vi "Test.vi"() -> ()   [LabVIEW 2019]
uses:
  <vilib>/NI/Modbus Library/API/Wrapper/Create Serial Master.vi
  <vilib>/NI/Modbus Library/API/Master/Modbus Master.lvclass
  <vilib>/NI/Modbus Library/API/Wrapper/API Main.lvlib
panel:
  in  "register to write":u16=50
  out "read values":u16[](array[numeric])
  in  "read count":u16=1
  in  "read starting address":u16=302 format="%04d"
  out "error out":errorcluster
  out "FTCU Input Reg Value":u16[](array[numeric])
  in  "FTCU Hold Reg Addr":u16=302 format="%04d"
  in  "FTCU Input Reg Addr":u16=8 format="%04d"
  in  "stop":bool
  in  "frequency":u16 caption="frequency, 0.01 Hz"
  in  "address":u16=895 format="%04x"
  in  "number of inputs":u16=1
  in  "starting address":u16=18 format="%04x"
  out "register values":u16[](array[numeric])
  # "G100"
  # "0h037F - adres zadawania prêdkoœci\ntab 7.6.2, str. 236"
  # "2 Hz to minimum"
  # "FTCU"
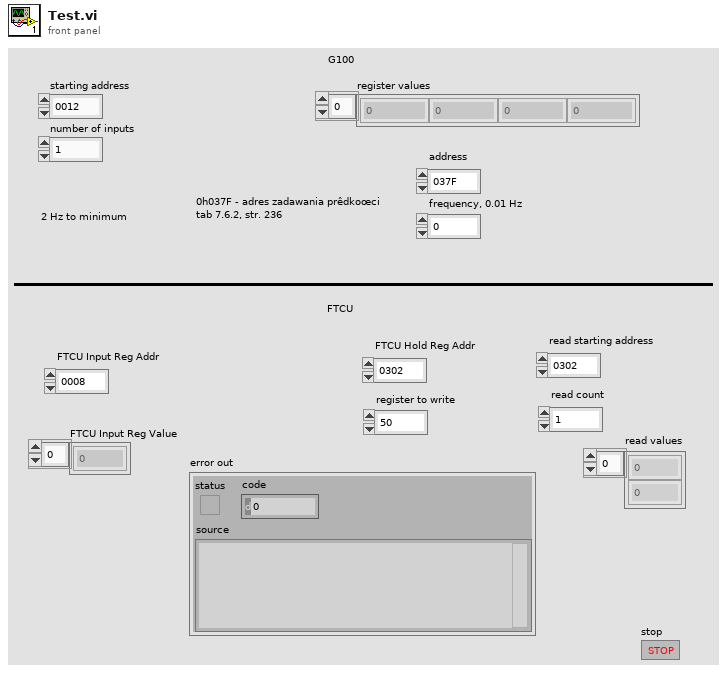
[diagram p1: front panel]
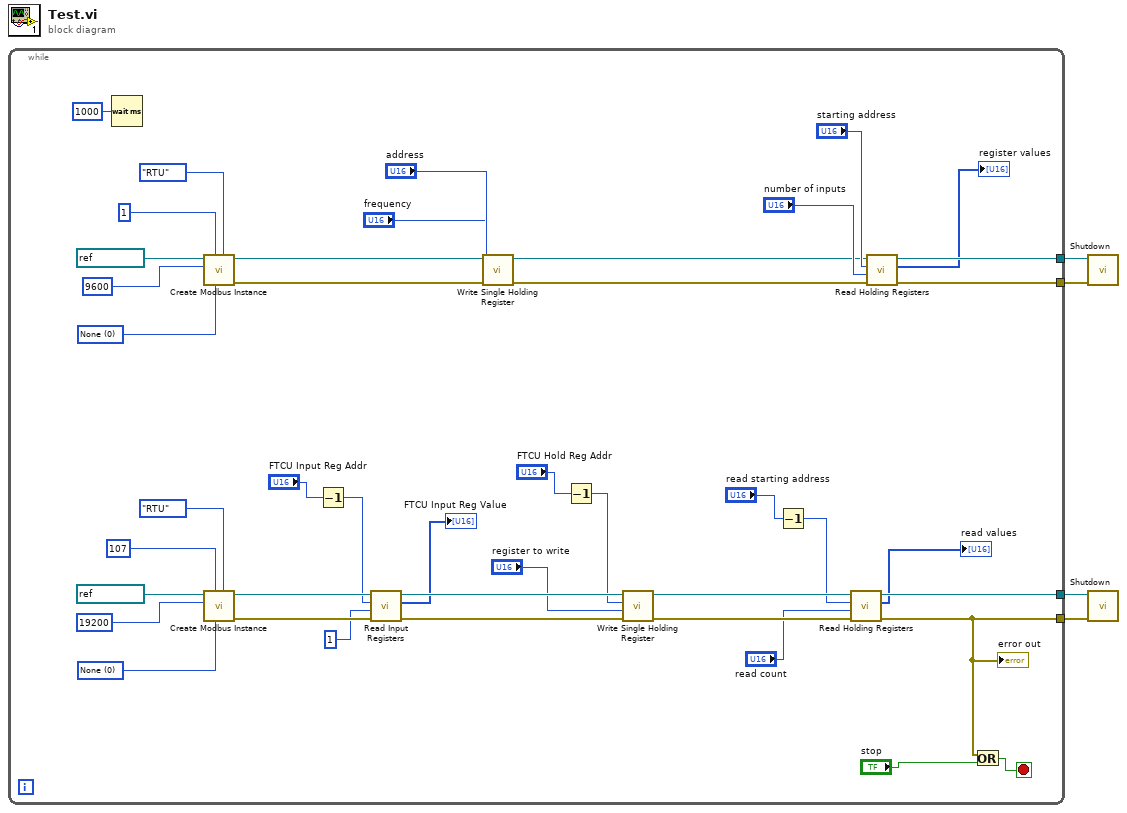
[diagram p0: block diagram]
diagram:
  n1 = while {
    tunnel: [w40] -> w4
    tunnel: [w39] -> w3
    tunnel: [w19] -> w1
    tunnel: [w17] -> w2
    stop <- w22 stop-if-true
    w28 = u16 0 items=["None", "Odd", "Even", "Mark", "Space"] ("parity (even)")
    w45 = u16 0 items=["None", "Odd", "Even", "Mark", "Space"] ("parity (even)")
    n2 = Wait (ms)(milliseconds to wait=u32 1000) -> ()  [unwired: 1 out]
    n3 = call-poly <vilib>:"Create Modbus Instance.vi"("serial type"=enum16{"RTU", "ASCII"}."RTU", "parity (even)"=w45, "unit ID"=u8 1, "baud rate"=u32 9600, "VISA resource name"=refnum<visa-resource-name> "COM21") -> ("error out"=w37:errorcluster, "serial master instance"=w36:refnum<class "Modbus Master.lvclass">)  [unwired: 5 in]
    n4 = call-poly <vilib>:"Create Modbus Instance.vi"("serial type"=enum16{"RTU", "ASCII"}."RTU", "parity (even)"=w28, "unit ID"=u8 107, "baud rate"=u32 19200, "VISA resource name"=refnum<visa-resource-name> "COM22") -> ("error out"=w24:errorcluster, "serial master instance"=w25:refnum<class "Modbus Master.lvclass">)  [unwired: 5 in]
    n5 = Decrement(x="FTCU Input Reg Addr") -> (x-1=w8:u16)
    n6 = call-dynamic "Read Input Registers.vi"("error in"=w24, "number of inputs"=u16 1, "starting address"=w8, "Modbus master in"=w25) -> ("error out"=w9:errorcluster, "register values"=→"FTCU Input Reg Value":u16[], "Modbus master out"=w11:refnum<class "Modbus Master.lvclass">)  [unwired: 5 in]
    n7 = call-dynamic "Write Single Holding Register.vi"("error in"=w37, "register to write"="frequency", "address"="address", "Modbus master in"=w36) -> ("error out"=w34:errorcluster, "Modbus master out"=w35:refnum<class "Modbus Master.lvclass">)  [unwired: 6 in]
    n8 = Decrement(x="FTCU Hold Reg Addr") -> (x-1=w6:u16)
    n9 = call-dynamic "Write Single Holding Register.vi"("error in"=w9, "register to write"="register to write", "address"=w6, "Modbus master in"=w11) -> ("error out"=w18:errorcluster, "Modbus master out"=w20:refnum<class "Modbus Master.lvclass">)  [unwired: 6 in]
    n10 = Decrement(x="read starting address") -> (x-1=w13:u16)
    n11 = call-dynamic "Read Holding Registers.vi"("error in"=w18, "number of inputs"="read count", "starting address"=w13, "Modbus master in"=w20) -> ("error out"=w17:errorcluster, "register values"=→"read values":u16[], "Modbus master out"=w19:refnum<class "Modbus Master.lvclass">)  [unwired: 5 in]
    "error out" <- w17
    n12 = call-dynamic "Read Holding Registers.vi"("error in"=w34, "number of inputs"="number of inputs", "starting address"="starting address", "Modbus master in"=w35) -> ("error out"=w40:errorcluster, "register values"=→"register values":u16[], "Modbus master out"=w39:refnum<class "Modbus Master.lvclass">)  [unwired: 5 in]
    n13 = Or(x=w17, y="stop") -> (x .or. y?=w22:bool)
  }
  n14 = call-dynamic "Shutdown.vi"("error in"=w4, "Modbus master in"=w3) -> ()  [unwired: 9 in, 1 out]
  n15 = call-dynamic "Shutdown.vi"("error in"=w2, "Modbus master in"=w1) -> ()  [unwired: 9 in, 1 out]
